vi "MultiplyDivideMarcoGonzalez.vi"() -> ()   [LabVIEW 2012]
panel:
  out "Greater Than Six":bool
  out "Operation Perform":string
  in  "?":bool
  in  "?":bool
  out "Z":dbl
  in  "Y":dbl
  in  "X":dbl
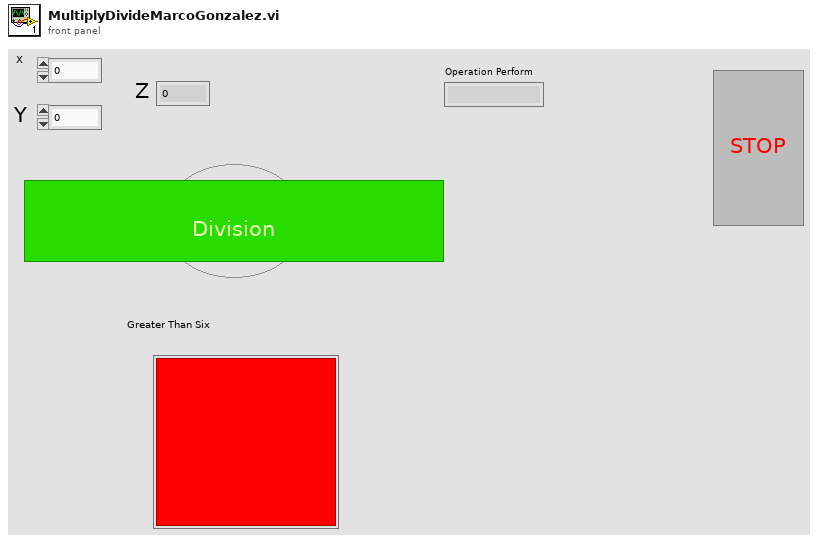
[diagram p1: front panel]
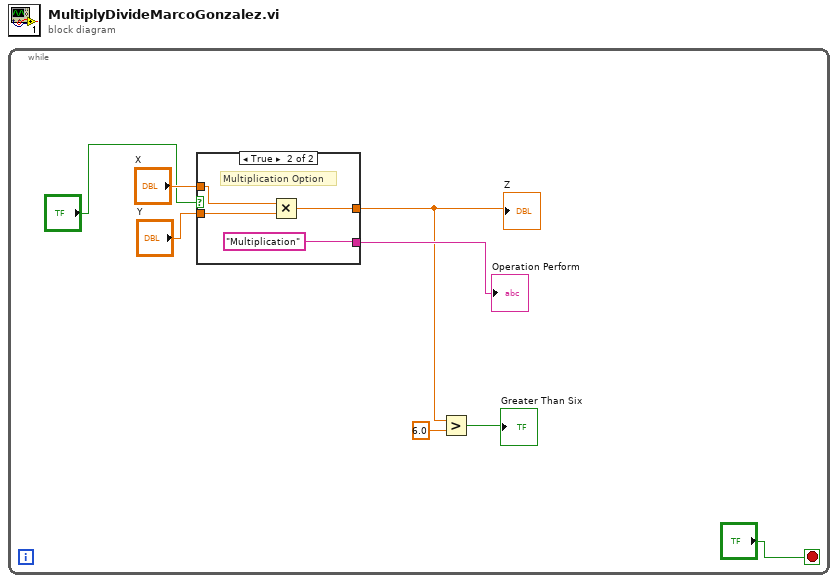
[diagram p0: block diagram]
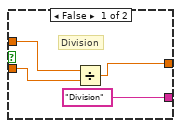
[diagram p2: hidden frame]
diagram:
  n1 = while {
    stop <- "?" stop-if-true
    n2 = case shown="True" "?" {
      tunnel: [w12 w16] -> w1
      tunnel: "X" -> [w11 w15]
      tunnel: "Y" -> [w10 w14]
      tunnel: ["Division" "Multiplication"] -> w4
      frame False {
        # "Division"
        n3 = Divide(x=w11, y=w10) -> (x/y=w12:dbl)
      }
      frame True {
        # "Multiplication Option"
        n4 = Multiply(x=w15, y=w14) -> (x*y=w16:dbl)
      }
    }
    "Z" <- w1
    "Operation Perform" <- w4
    n5 = Greater?(x=w1, y=6.0) -> (0:→"Greater Than Six":bool)
  }
